vi "Get Sync Data.vi"(8 "error in (no error)":errorcluster, 11 "Filled Text Fields Actor in":refnum<class "Filled Text Fields Actor.lvclass">) -> (0 "error out":errorcluster, 1 "Theme":refnum<class "Theme.lvclass">, 2 "Data":refnum<class "Data.lvclass">, 3 "Filled Text Fields Actor out":refnum<class "Filled Text Fields Actor.lvclass">)   [LabVIEW 2017, in "Filled Text Fields.lvlib" / "Filled Text Fields Actor.lvclass"]
uses:
  Filled Text Fields Actor.lvclass
  Theme/Theme/Theme.lvclass
  Data/Data.lvclass
  Filled Text Fields Actor.lvclass/Filled Text Fields Actor.ctl
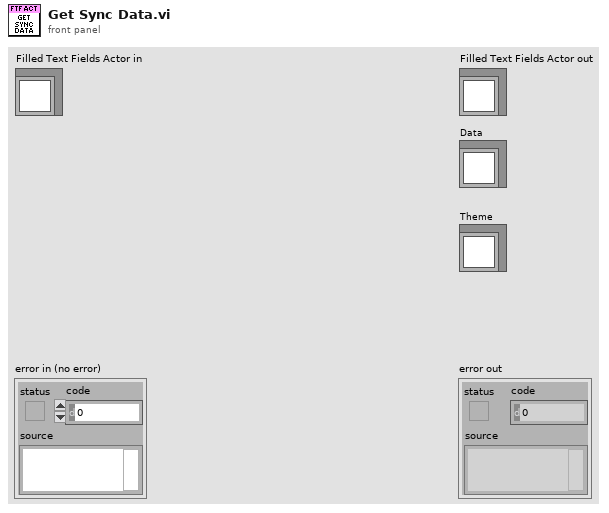
[diagram p1: front panel]
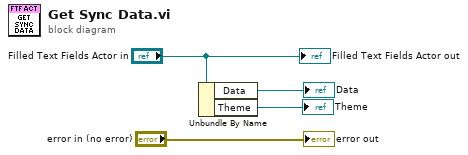
[diagram p0: block diagram]
diagram:
  n1 = Unbundle By Name("Filled Text Fields Actor in") -> ("Data"=→"Data":refnum<class "Data.lvclass">, "Theme"=→"Theme":refnum<class "Theme.lvclass">)
  "error out" <- "error in (no error)"
  "Filled Text Fields Actor out" <- "Filled Text Fields Actor in"
